vi "Lock in Voltage measurement.vi"(7 "Stanford Error In":errorcluster, 10 "Stanford ID":refnum<visa-resource-name>) -> (0 "error out":errorcluster, 2 "Voltage-Value":dbl, 3 "Reference Frequency":dbl)   [LabVIEW 2013]
doc: "This example shows how to configure the instrument to read all the parameters available."
uses:
  <instrlib>/Stanford Research 830/Public/Data/Read (All Parameters).vi
  <instrlib>/Stanford Research 830/Stanford Research 830.lvlib
panel:
  # "(c) 2006 National Instruments.  ALL RIGHTS RESERVED."
  # "READOUT"
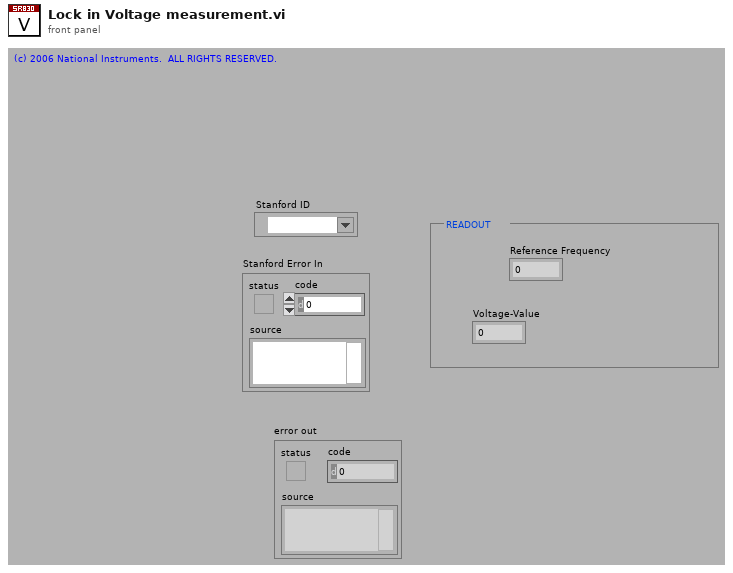
[diagram p1: front panel]
types:
  T1 = cluster{"X-Value":dbl, "Y-Value":dbl, "R-Value":dbl, "Theta-Value":dbl, "Aux In 1 Value":dbl, "Aux In 2 Value":dbl, "Aux In 3 Value":dbl, "Aux In 4 Value":dbl, "Reference Frequency":dbl, "Channel 1 Display":dbl, "Channel 2 Display":dbl}
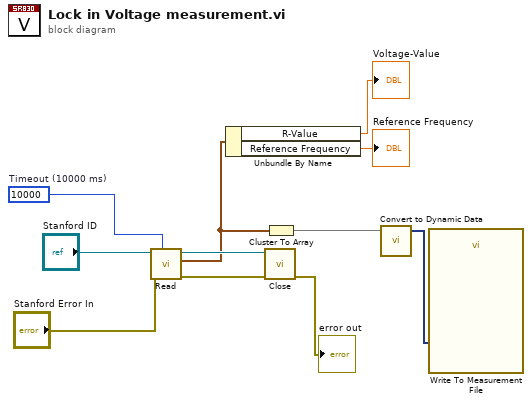
[diagram p0: block diagram]
diagram:
  w8 = u32 10000  # Timeout (10000 ms)
  n1 = call-poly <instrlib>:"Read.vi"("Timeout (10000 ms)"=w8, "error in (no error)"="Stanford Error In", "VISA resource name"="Stanford ID") -> ("error out"=w9:errorcluster, "Parameter Values"=w5:T1, "VISA resource name out"=w10:refnum<visa-resource-name>)  [unwired: 6 in]
  n2 = Unbundle By Name(w5) -> ("R-Value"=→"Voltage-Value":dbl, "Reference Frequency"=→"Reference Frequency":dbl)
  n3 = call <instrlib>:"Close.vi"("error in (no error)"=w9, "VISA resource name"=w10) -> ("error out"=→"error out":errorcluster)  [unwired: 9 in]
  n4 = Cluster To Array(cluster=w5) -> (array=w7:dbl[])
  n5 = call "Convert to Dynamic Data"("Array"=w7) -> ("Dynamic Data Type"=w6:dynamicdata)  [unwired: 3 in]
  n6 = call "Write To Measurement File"("Signals"=w6) -> ()  [unwired: 16 in, 3 out]
